vi "check_styx_null.vi"(0 "error in (no error)":errorcluster, 3 "ptr":u32) -> (2 "error out":errorcluster)   [LabVIEW 2010, in "lib1299.lvlib"]
uses:
  lib1299.lvlib
  cstyx/win32/cstyx.dll
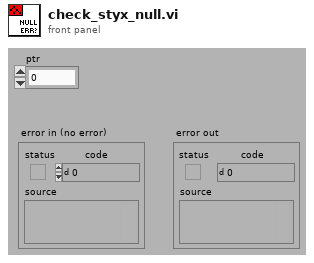
[diagram p1: front panel]
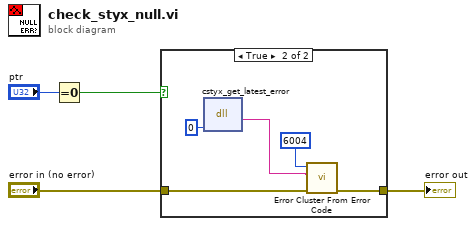
[diagram p0: block diagram]
diagram:
  n1 = Equal To 0?(x="ptr") -> (x = 0?=w2:bool)
  n2 = case shown="True" w2 {
    tunnel: [w5 w9] -> w4
    tunnel: "error in (no error)" -> [w5 w8]
    frame False {
    }
    frame True {
      n3 = dll-call lib="C:/work/ads1299evm/lib_1299/Styx/cstyx/win32/cstyx.dll" fn="cstyx_get_latest_error"("code"=0) -> (w6:string)  [unwired: 4 in, 2 out]
      n4 = call <vilib>:"Error Cluster From Error Code.vi"("error in (no error)"=w8, "error message (\"\")"=w6, "error code (0)"=6004 ("[error code] (0)")) -> ("error out"=w9:errorcluster)  [unwired: 6 in]
    }
  }
  "error out" <- w4
